vi "AskForExperimentDescription.vi"(7 "String Control":string) -> (0 "Disable Button 2":bool, 1 "Experiment Name 2":string)   [LabVIEW 2024]
panel:
  in  "Disable Button":bool
  in  "OK Button":bool
  in  "Experiment Description":string
  # "Please describe the experiment you are performing."
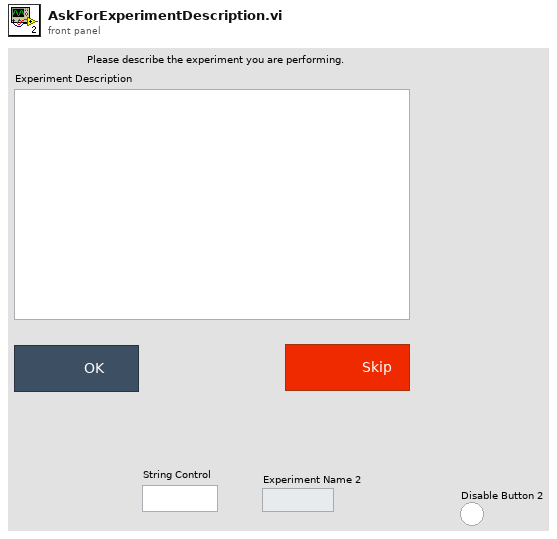
[diagram p1: front panel]
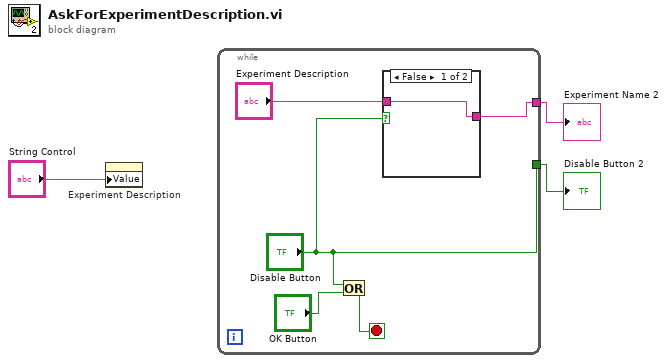
[diagram p0: block diagram]
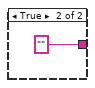
[diagram p2: hidden frame]
diagram:
  n1 = property on="Experiment Description" class="Str"("Value"="String Control") -> ()  [unwired: 2 in, 2 out]
  n2 = while {
    tunnel: [w5] -> w2
    tunnel: ["Disable Button"] -> w1
    stop <- w7 stop-if-true
    n3 = Or(x="Disable Button", y="OK Button") -> (x .or. y?=w7:bool)
    n4 = case shown="False" "Disable Button" {
      tunnel: [w9 "" ("Experiment Description")] -> w5
      tunnel: "Experiment Description" -> [w9 _]
      frame False {
      }
      frame True {
      }
    }
  }
  "Experiment Name 2" <- w2
  "Disable Button 2" <- w1
